vi "Forebrain Lidar Functional Global.vi"(2 "Lidar Angle Data In (Degrees)":sgl[](array[numeric]), 3 "Lidar Magnitude Data In (mm)":sgl[](array[numeric]), 4 "Lidar Action":enum16{"Set Lidar Data", "Read Lidar Data"}(ring)) -> (0 "Lidar Angle Data Out (Degrees)":sgl[](array[numeric]), 1 "Lidar Magnitude Data Out (mm)":sgl[](array[numeric]))   [LabVIEW 2011]
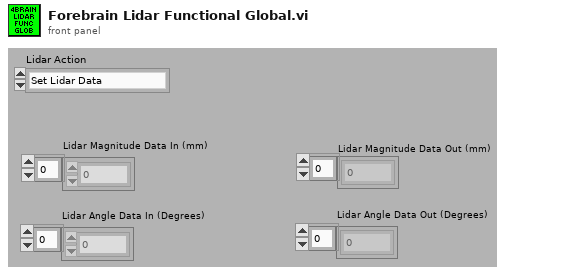
[diagram p1: front panel]
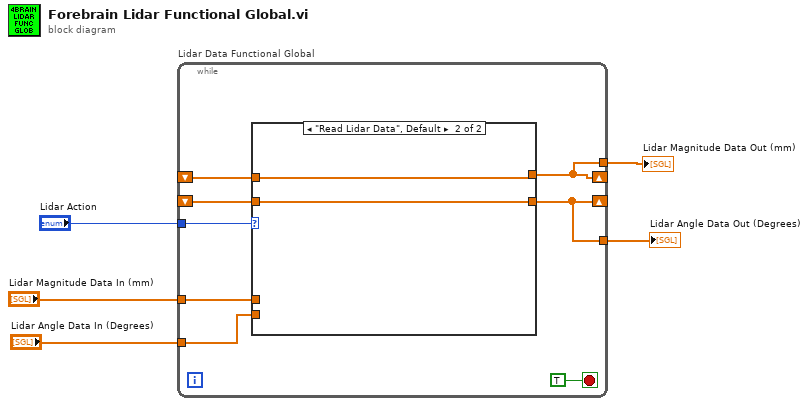
[diagram p0: block diagram]
diagram:
  n1 = while "Lidar Data Functional Global" {
    shift-right: [w6] -> _
    shift-left: _ -> [w10]
    tunnel: "Lidar Action" -> [w13]
    shift-right: [w7] -> _
    shift-left: _ -> [w9]
    tunnel: "Lidar Angle Data In (Degrees)" -> [w12]
    tunnel: "Lidar Magnitude Data In (mm)" -> [w11]
    tunnel: [w7] -> w2
    tunnel: [w6] -> w1
    stop <- TRUE stop-if-true
    n2 = case shown="\"Read Lidar Data\", Default" w13 {
      tunnel: [w15 w16] -> w7
      tunnel: w12 -> [w15 _]
      tunnel: [w14 w17] -> w6
      tunnel: w11 -> [w14 _]
      tunnel: w10 -> [_ w17]
      tunnel: w9 -> [_ w16]
      frame "Set Lidar Data" {
      }
      frame "Read Lidar Data", Default {
      }
    }
  }
  "Lidar Angle Data Out (Degrees)" <- w2
  "Lidar Magnitude Data Out (mm)" <- w1
